vi "NI 9425_TASK_DI.vi"(8 "error in":errorcluster, 11 "MODULE NAME":string="cDAQ_NICOTRAMod1") -> (0 "error out":errorcluster, 3 "task out":refnum<k21>)   [LabVIEW 2016]
uses:
  <vilib>/DAQmx/create/channels.llb/DAQmx Create Channel (DI-Digital Input).vi
  <resource>/objmgr/daqmx.rc
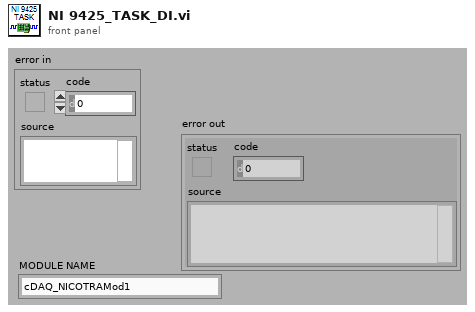
[diagram p1: front panel]
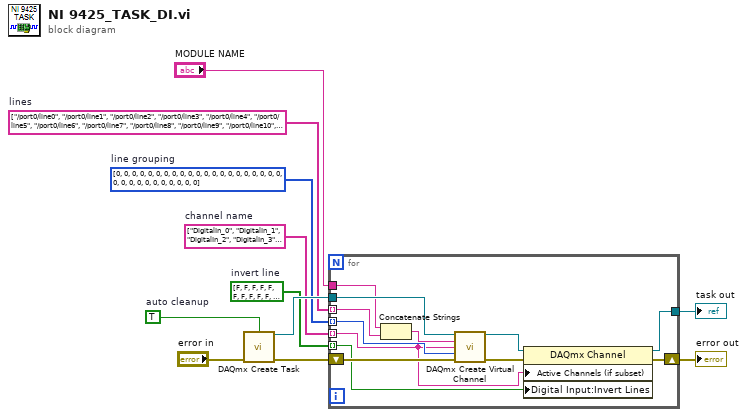
[diagram p0: block diagram]
diagram:
  w7 = bool[] [FALSE, FALSE, FALSE, FALSE, FALSE, FALSE, FALSE, FALSE, FALSE, FALSE, FALSE, FALSE, FALSE, FALSE, FALSE, FALSE, FALSE, FALSE, FALSE, FALSE, FALSE, FALSE, FALSE, FALSE, FALSE, FALSE, FALSE, FALSE, FALSE, FALSE, FALSE, FALSE]  # invert line
  w6 = i32[] [0, 0, 0, 0, 0, 0, 0, 0, 0, 0, 0, 0, 0, 0, 0, 0, 0, 0, 0, 0, 0, 0, 0, 0, 0, 0, 0, 0, 0, 0, 0, 0] items=["one channel for each line", "one channel for all lines"]  # line grouping
  w5 = string[] ["DigitalIn_0", "DigitalIn_1", "DigitalIn_2", "DigitalIn_3", "DigitalIn_4", "DigitalIn_5", "DigitalIn_6", "DigitalIn_7", "DigitalIn_8", "DigitalIn_9", "DigitalIn_10", "DigitalIn_11", "DigitalIn_12", "DigitalIn_13", "DigitalIn_14", "DigitalIn_15", "DigitalIn_16", "DigitalIn_17", "DigitalIn_18", "DigitalIn_19", "DigitalIn_20", "DigitalIn_21", "DigitalIn_22", "DigitalIn_23", "DigitalIn_24", "DigitalIn_25", "DigitalIn_26", "DigitalIn_27", "DigitalIn_28", "DigitalIn_29", "DigitalIn_30", "DigitalIn_31"]  # channel name
  w4 = string[] ["/port0/line0", "/port0/line1", "/port0/line2", "/port0/line3", "/port0/line4", "/port0/line5", "/port0/line6", "/port0/line7", "/port0/line8", "/port0/line9", "/port0/line10", "/port0/line11", "/port0/line12", "/port0/line13", "/port0/line14", "/port0/line15", "/port0/line16", "/port0/line17", "/port0/line18", "/port0/line19", "/port0/line20", "/port0/line21", "/port0/line22", "/port0/line23", "/port0/line24", "/port0/line25", "/port0/line26", "/port0/line27", "/port0/line28", "/port0/line29", "/port0/line30", "/port0/line31"]  # lines
  w9 = TRUE  # auto cleanup
  n1 = call <vilib>:"DAQmx Create Task.vi"("auto cleanup"=w9, "error in"="error in") -> ("task out"=w8:refnum<k21>, "error out"=w10:errorcluster)  [unwired: 12 in]
  n2 = for {
    tunnel: w8 -> [w23]
    tunnel: w7 -> [w18] mode=indexing
    tunnel: w6 -> [w21] mode=indexing
    tunnel: w5 -> [w17] mode=indexing
    tunnel: w4 -> [w14] mode=indexing
    tunnel: [w19] -> w3
    shift-right: [w15] -> w2
    shift-left: w10 -> [w22]
    tunnel: "MODULE NAME" -> [w13]
    n3 = Concatenate Strings(w13, w14) -> (w12:string)
    n4 = call-poly <vilib>:"DAQmx Create Virtual Channel.vi"("task in"=w23, "lines"=w12, "name to assign"=w17, "line grouping"=w21, "error in"=w22) -> ("task out"=w20:refnum<k21>, "error out"=w16:errorcluster)  [unwired: 9 in]
    n5 = property class="DAQmx Channel"(reference=w20, error in=w16, "Active Channels (if subset)"=w17, "Digital Input:Invert Lines"=w18) -> (reference out=w19:refnum<k21>, error out=w15:errorcluster)
  }
  "error out" <- w2
  "task out" <- w3
